vi "20170502-lecture4-1 write labview measurement file (merge signal).vi"   [LabVIEW 2014]
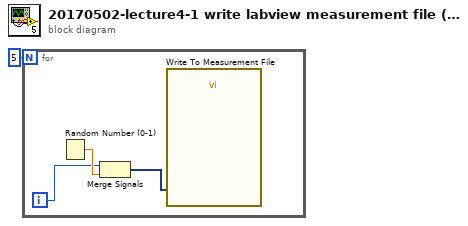
[diagram p0: block diagram]
diagram:
  n1 = for {
    N: 5 -> [_]
    i -> [w2]
    n2 = Random Number (0-1)() -> (number: 0 to 1=w3:dbl)
    n3 = Merge Signals(w2, w3) -> (w4:dynamicdata)
    n4 = call "Write To Measurement File"("Signals"=w4) -> ()  [unwired: 16 in, 3 out]
  }
